vi "Loop_UpDownACT.vi"() -> ()   [LabVIEW 2017, in "Gimbal.lvlib"]
uses:
  Gimbal.lvlib
  <vilib>/Rock Robotics/SystemInterfaces/DIO/FPGA_DIOPWMChannel.ctl
  _SHARE ALL/Global Share All/Global_STOP.vi
  Global_SM Write_Data Out.vi
  Global_ACT Write_Data Out.vi
panel:
  out "Output Data":dbl
  out "Input Data":dbl
  out "Cycle Time (S)":dbl format="%.3g"
  in  "Target Time(ms)":u32=50
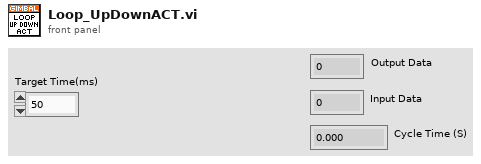
[diagram p1: front panel]
types:
  T1 = typedef "FPGA_DIOPWMChannel.ctl" = enum8{"PWM 0", "PWM 1", "PWM 2", "PWM 3", "PWM 4", "PWM 5", "PWM 6", "PWM 7", "PWM 8", "PWM 9", "PWM MXP 0", "PWM MXP 1", "PWM MXP 2", "PWM MXP 3", "PWM MXP 4", "PWM MXP 5", "PWM MXP 6", "PWM MXP 7", "PWM MXP 8", "PWM MXP 9", "Invalid"}
  T2 = typedef "WPI_ServoDeviceRef.ctl" = cluster{"DeviceStatus":errorcluster, "PWM Channel":T1, "DeadBand":T3}
  T3 = typedef "WPI_PWMDeadband.ctl" = cluster{"Name":string, "maxPositivePwm":i32, "minPositivePwm":i32, "centerPwm":i32, "maxNegativePwm":i32, "minNegativePwm":i32, "angularRange":u16}
  T4 = cluster{"ServoDeviceRef":T2, " Angle Output":i32, "Angle Input":i32, "Target Time(ms)":u32, "Current Time":timestamp, "Previous Time":timestamp, "Cycle Time (S)":dbl}
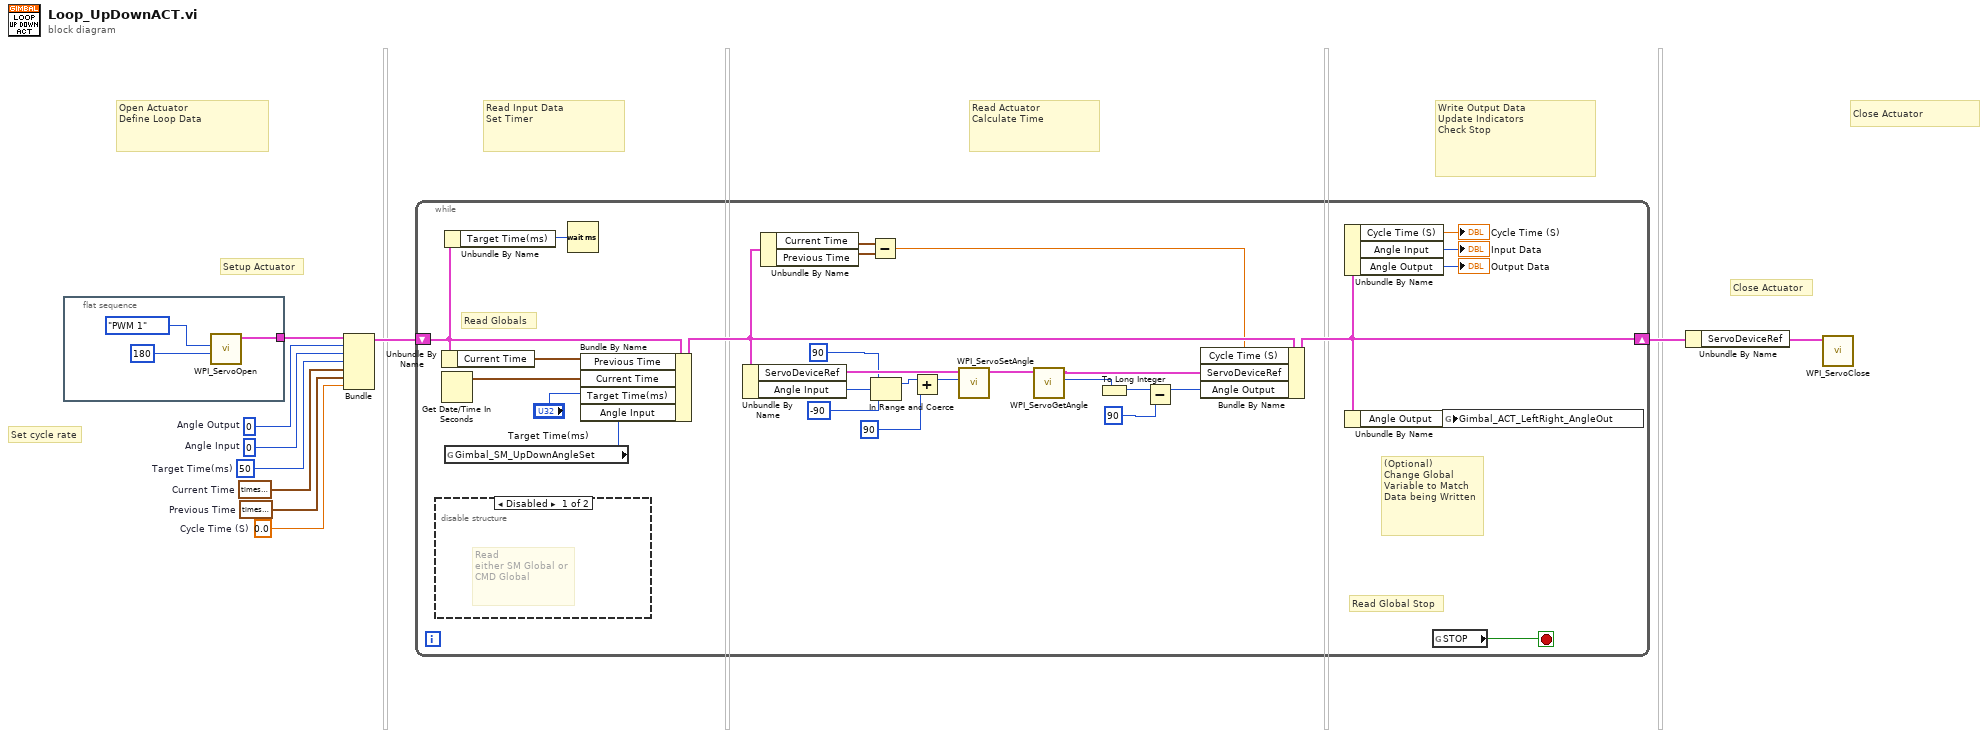
[diagram p0: block diagram]
diagram:
  w2 = 0.0  # Cycle Time (S)
  w10 = timestamp(0 s since 1904-01-01)  # Previous Time
  w9 = timestamp(0 s since 1904-01-01)  # Current Time
  w8 = u32 50  # Target Time(ms)
  w7 = 0  # Angle Input
  w5 = 0  # Angle Output
  # "Close Actuator"
  # "Write Output Data\nUpdate Indicators\nCheck Stop"
  # "Read Actuator\nCalculate Time"
  # "Read Input Data\nSet Timer"
  # "Open Actuator\nDefine Loop Data"
  # "Set cycle rate"
  # "Close Actuator"
  # "Setup Actuator"
  n1 = flat-sequence {
    tunnel: [w12] -> w4
    frame #0 {
      n2 = call <vilib>:"WPI_ServoOpen.vi"("Angular Range"=u16 180, "PWM Channel"=FPGA_DIOPWMChannel."PWM 1") -> ("ServoDeviceRef"=w12:T2)  [unwired: 2 in, 7 out]
    }
  }
  n3 = Bundle("ServoDeviceRef"=w4, "Angle Output"=w5, "Angle Input"=w7, "Target Time(ms)"=w8, "Current Time"=w9, "Previous Time"=w10, "Cycle Time (S)"=w2) -> (w6:T4)  [unwired: 1 in]
  n4 = while {
    shift-right: [w33] -> w3
    shift-left: w6 -> [w35]
    stop <- w42 stop-if-true
    # "(Optional)\nChange Global\nVariable to Match\nData being Written"
    # "Read Globals"
    # "Read Global Stop"
    n5 = disable-structure shown="Disabled" {
      frame Disabled {
        # "Read\neither SM Global or CMD Global"
      }
      frame Enabled {
      }
    }
    n6 = Unbundle By Name(w35) -> ("Current Time"=w40:timestamp)
    n7 = Get Date/Time In Seconds() -> (seconds since 1Jan1904=w41:timestamp)
    n8 = Unbundle By Name(w35) -> ("Target Time(ms)"=w34:u32)
    n9 = global read "Global_SM Write_Data Out.vi" "Gimbal_SM_UpDownAngleSet"() -> (w16:i32)
    n10 = Wait (ms)(milliseconds to wait=w34) -> ()  [unwired: 1 out]
    n11 = Bundle By Name(cluster=w35, "Previous Time"=w40, "Current Time"=w41, "Target Time(ms)"="Target Time(ms)", "Angle Input"=w16) -> (w36:T4)
    n12 = Unbundle By Name(w36) -> ("ServoDeviceRef"=w27:T2, "Angle Input"=w22:i32)
    n13 = Unbundle By Name(w36) -> ("Current Time"=w39:timestamp, "Previous Time"=w38:timestamp)
    n14 = Subtract(x=w39, y=w38) -> (x-y=w29:dbl)
    n15 = In Range and Coerce(upper limit=90, x=w22, lower limit=-90 ("upper limit")) -> (coerced(x)=w21:i32)  [unwired: 1 out]
    n16 = Add(x=w21, y=90) -> (x+y=w18:i32)
    n17 = call <vilib>:"WPI_ServoSetAngle.vi"("Angle"=w18, "ServoDeviceRef"=w27) -> ("ServoDeviceRef"=w26:T2)  [unwired: 1 in, 8 out]
    n18 = call <vilib>:"WPI_ServoGetAngle.vi"("ServoDeviceRef"=w26) -> ("ServoDeviceRef"=w25:T2, "Angle"=w24:u16)  [unwired: 1 in, 7 out]
    n19 = To Long Integer(number=w24) -> (32bit integer=w23:i32)
    n20 = Subtract(x=w23, y=90) -> (x-y=w15:i32)
    n21 = Bundle By Name(cluster=w36, "Cycle Time (S)"=w29, "ServoDeviceRef"=w25, "Angle Output"=w15) -> (w33:T4)
    n22 = Unbundle By Name(w33) -> ("Cycle Time (S)"=→"Cycle Time (S)":dbl, "Angle Input"=→"Input Data":i32, "Angle Output"=→"Output Data":i32)
    n23 = Unbundle By Name(w33) -> ("Angle Output"=w28:i32)
    n24 = global read "Global_STOP.vi" "STOP"() -> (w42:bool)
    n25 = global write "Global_ACT Write_Data Out.vi" "Gimbal_ACT_LeftRight_AngleOut"(w28) -> ()
  }
  n26 = Unbundle By Name(w3) -> ("ServoDeviceRef"=w1:T2)
  n27 = call <vilib>:"WPI_ServoClose.vi"("ServoDeviceRef"=w1) -> ()  [unwired: 1 in, 10 out]
